vi "LoadTWPValues.vi"(8 "error in (no error)":errorcluster) -> (0 "error out":errorcluster)   [LabVIEW 2015]
uses:
  Drive/Implementation/Advanced Drive VIs/PID Type Def.ctl
  Port/PortC Settings Type Def.ctl
  <vilib>/Rock Robotics/Network Tables/NT Read Numeric Array.vi
  Lift/TW Global.vi
panel:
  out "Settings":T1={"Down"=-230.0, "Up"=140.0, "Increments"=-230.0, "Final Pos"=-230.0}
  out "PID":T2
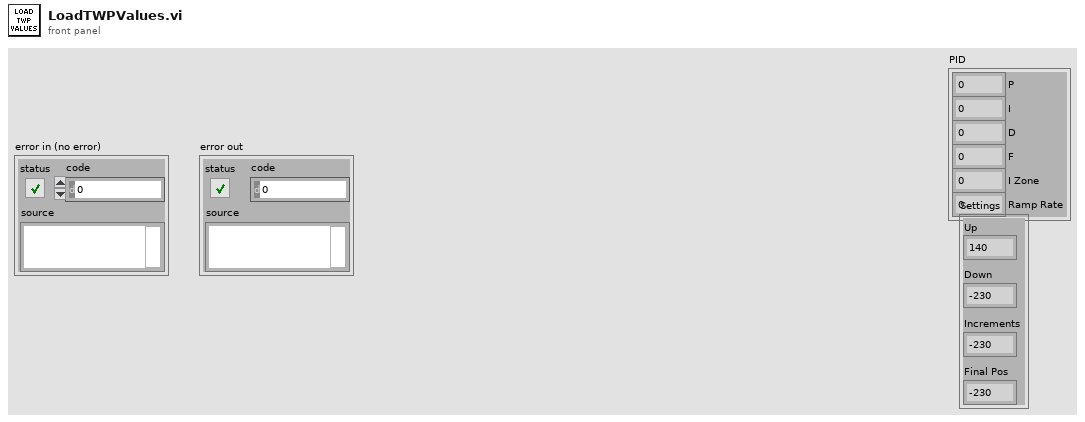
[diagram p1: front panel]
types:
  T1 = typedef "PortC Settings Type Def.ctl" = cluster{"Down":dbl, "Up":dbl, "Increments":dbl, "Final Pos":dbl}
  T2 = typedef "PID Type Def.ctl" = cluster{"P":dbl, "I":dbl, "D":dbl, "F":dbl, "I Zone":dbl, "Ramp Rate":dbl}
  T3 = typedef "Detailed Motor Type Def.ctl" = cluster{"MotorRef":T4, "Encoder Ticks Per Rev":dbl, "Set Position":dbl, "Wheel Radius":dbl}
  T4 = typedef "WPI_MotorControlDeviceRef.ctl" = cluster{"DeviceStatus":errorcluster, "Type":T5, "PWM":cluster{"PWM Channel":T6, "DeadBand":T7}, "CAN":cluster{"Device Number":u8, "Control Mode":T8, "Semaphore":T9, "Max Vout":dbl, "TalonSRX Control Mode":T10}, "Invert":bool}
  T5 = typedef "WPI_MotorControlType.ctl" = enum16{"PWM", "CAN", "CANTalonSRX"}
  T6 = typedef "FPGA_DIOPWMChannel.ctl" = enum8{"PWM 0", "PWM 1", "PWM 2", "PWM 3", "PWM 4", "PWM 5", "PWM 6", "PWM 7", "PWM 8", "PWM 9", "PWM MXP 0", "PWM MXP 1", "PWM MXP 2", "PWM MXP 3", "PWM MXP 4", "PWM MXP 5", "PWM MXP 6", "PWM MXP 7", "PWM MXP 8", "PWM MXP 9", "Invalid"}
  T7 = typedef "WPI_PWMDeadband.ctl" = cluster{"Name":string, "maxPositivePwm":i32, "minPositivePwm":i32, "centerPwm":i32, "maxNegativePwm":i32, "minNegativePwm":i32, "angularRange":u16}
  T8 = typedef "WPI_CANJaguar_ControlMode.ctl" = enum8{"Percent VBus", "Current", "Speed", "Position", "Voltage"}
  T9 = typedef "Semaphore RefNum" = refnum<k1>
  T10 = typedef "WPI_CANTalonSRX_APIControlMode.ctl" = enum8{"Percent VBus", "Speed", "Position", "Slave", "Unchanged / Invalid", "Voltage Compensation", "Current", "Motion Profile"}
  T11 = typedef "WPI_CANTalonSRX_GlobalStatus.ctl" = cluster{"Applied Throttle":dbl, "Module Enabled":bool, "CAN Error":errorcluster, "Closed Loop Error":dbl, "Forward Limit Switch Closed":bool, "Reverse Limit Switch Closed":bool, "Sensor Position":dbl, "Sensor Velocity":dbl, "Current":dbl, "Sticky Fault - Over Temp":bool, "Sticky Fault - Under Voltage":bool, "Sticky Fault - Forward Limit":bool, "Sticky Fault - Reverse Limit":bool, "Sticky Fault - Forward Soft Limit":bool, "Sticky Fault - Reverse Soft Limit":bool, "Brake is Enabled":bool, "Encoder Position":dbl, "Encoder Velocity":dbl, "Encoder Index Count":dbl, "Encoder A Pin State":bool, "Encoder B Pin State":bool, "Encoder Index Pin State":bool, "Analog In":dbl, "Analog In Velocity":dbl, "Temperature (C)":dbl, "Battery Voltage":dbl, "Control 5 Is Supported":bool, "Current Profile Slot Select":dbl, "Pos Div 8":bool, "Vel Div 4":bool, "Pulse Width Position":i32, "Pulse Width Velocity":i32, "Pulse Width Rise To Rise (us)":i32, "Pulse Width Rise To Fall (us)":i32, "Mot Prof Active Is Under Run":bool, "Mot Prof Active Has Under Run":bool, "Mot Prof Active Is Last":bool, "Mot Prof Active Velocity Only":bool, "Mot Prof Active Is Valid":bool, "Mot Prof Buffer Is Full":bool, "Mot Prof Active Profile Slot Select":i32, "Mot Prof NextID":i32, "Mot Prof Count":i32, "Mot Prof Active Velocity":dbl, "Mot Prof Active Position":dbl, "Mot Prof Output Enable":i32}
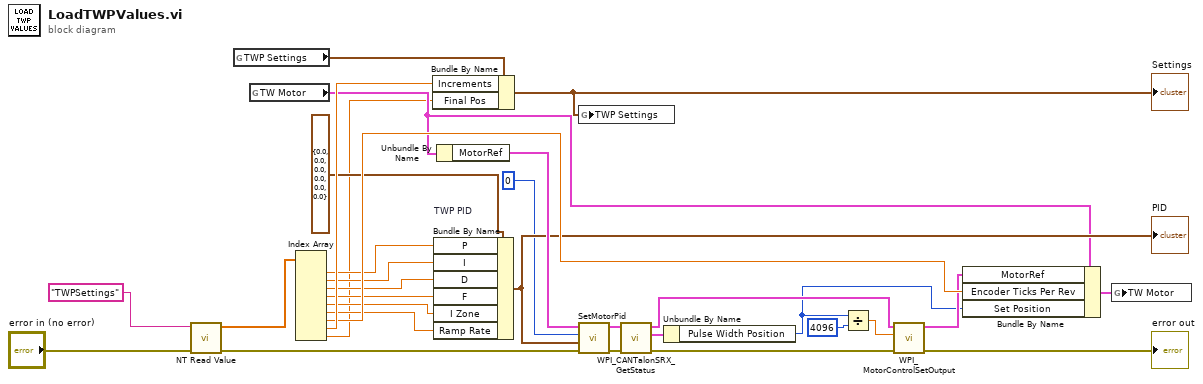
[diagram p0: block diagram]
diagram:
  n1 = call-poly <vilib>:"NT Read Value.vi"("error in"="error in (no error)", "Name"="TWPSettings") -> ("error out"=w17:errorcluster, "Numeric Array"=w21:dbl[])  [unwired: 8 in]
  n2 = global read "TW Global.vi" "TWP Settings"() -> (w15:T1)
  n3 = global read "TW Global.vi" "TW Motor"() -> (w14:T3)
  n4 = Index Array(array=w21) -> (element #1=w22:dbl, element #2=w23:dbl, element #3=w24:dbl, element #4=w25:dbl, element #5=w26:dbl, element #6=w27:dbl, element #7=w29:dbl, element #8=w30:dbl, element #9=w11:dbl)  [unwired: 9 in]
  n5 = Bundle By Name(cluster=w15, "Increments"=w30, "Final Pos"=w11) -> (w16:T1)
  "Settings" <- w16
  n6 = Bundle By Name "TWP PID"(cluster=T2 {"P"=0.0, "I"=0.0, "D"=0.0, "F"=0.0, "I Zone"=0.0, "Ramp Rate"=0.0} ("PID"), "P"=w22, "I"=w23, "D"=w24, "F"=w25, "I Zone"=w26, "Ramp Rate"=w27) -> (w28:T2)
  "PID" <- w28
  n7 = Unbundle By Name(w14) -> ("MotorRef"=w31:T4)
  n8 = global write "TW Global.vi" "TWP Settings"(w16) -> ()
  n9 = call "SetMotorPid.vi"("error in (no error)"=w17, "PID"=w28, "Parameter Slot"=u8 0, "Motor Ref In"=w31) -> ("error out"=w3:errorcluster, "Motor Ref Out"=w6:T4)  [unwired: 6 in]
  n10 = call <vilib>:"WPI_CANTalonSRX_GetStatus.vi"("error in (no error)"=w3, "CAN Talon SRX Ref"=w6) -> ("error out"=w8:errorcluster, "Talon SRX Status"=w7:T11, "CAN Talon SRX Ref"=w5:T4)  [unwired: 7 in]
  n11 = Unbundle By Name(w7) -> ("Pulse Width Position"=w1:i32)
  n12 = Divide(x=w1, y=4096) -> (x/y=w9:dbl)
  n13 = call <vilib>:"WPI_MotorControlSetOutput.vi"("error in (no error)"=w8, "Output"=w9, "MotorControlDevRef"=w5) -> ("error out"=→"error out":errorcluster, "MotorControlDevRef"=w4:T4)  [unwired: 6 in, 1 out]
  n14 = Bundle By Name(cluster=w14, "MotorRef"=w4, "Encoder Ticks Per Rev"=w29, "Set Position"=w1) -> (w13:T3)
  n15 = global write "TW Global.vi" "TW Motor"(w13) -> ()
